vi "ExtraDownsample_4channel.vi"(6 "reset":bool, 7 "Set downsample":bool, 8 "valid in":bool, 9 "Downsample":fxp<+,8,8>, 10 "CIC Gain":fxp<+/-,32,1>=0.00390625 format="%#_32g", 11 "Data in":fxp<+/-,16,14>[](array[numeric])=[0.0, 0.0, 0.0, 0.0, 0.0, 0.0, 0.0, 0.0]) -> (0 "valid out":bool, 3 "Data out":fxp<+/-,16,14>[](array[numeric]))   [LabVIEW 2013]
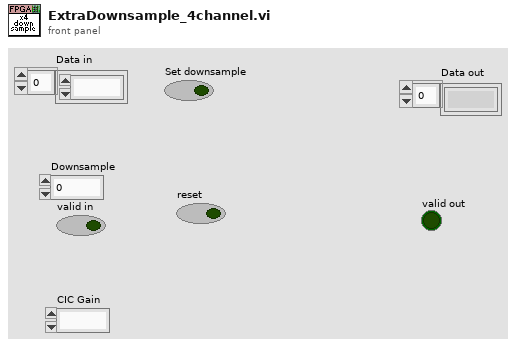
[diagram p1: front panel]
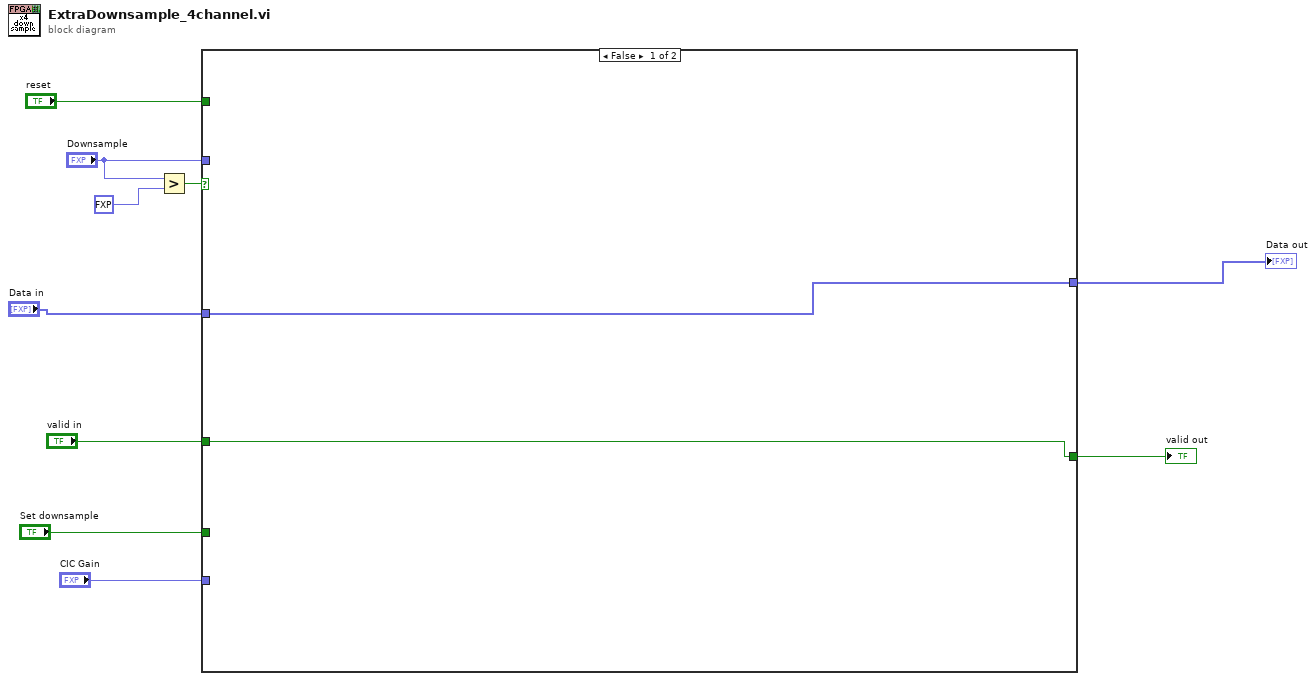
[diagram p0: block diagram]
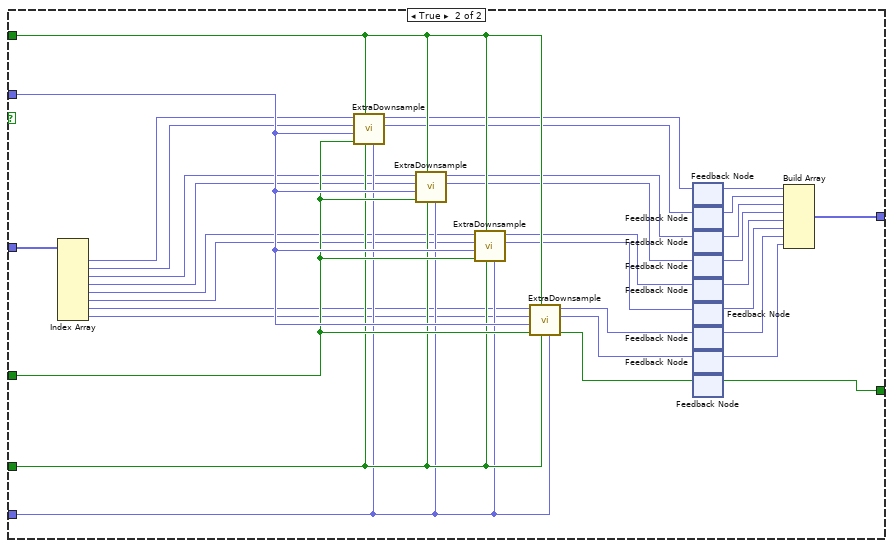
[diagram p2: hidden frame]
diagram:
  n1 = Greater?(x="Downsample", y=fxp<+,8,8> 1.0) -> (0:w2:bool)
  n2 = case shown="False" w2 {
    tunnel: "Data in" -> [w11 w45]
    tunnel: "Downsample" -> [_ w44]
    tunnel: "valid in" -> [w12 w43]
    tunnel: "reset" -> [_ w42]
    tunnel: "Set downsample" -> [_ w41]
    tunnel: "CIC Gain" -> [_ w40]
    tunnel: [w12 w30] -> w3
    tunnel: [w11 w13] -> w1
    frame False {
    }
    frame True {
      n3 = Index Array(array=w45) -> (element #1=w29:fxp<+/-,16,14>, element #2=w28:fxp<+/-,16,14>, element #3=w27:fxp<+/-,16,14>, element #4=w26:fxp<+/-,16,14>, element #5=w25:fxp<+/-,16,14>, element #6=w24:fxp<+/-,16,14>, element #7=w23:fxp<+/-,16,14>, element #8=w22:fxp<+/-,16,14>)  [unwired: 8 in]
      n4 = call "ExtraDownsample.vi"("CIC Gain"=w40, "Set downsample"=w41, "reset"=w42, "valid in"=w43, "Downsample"=w44, "I in"=w28, "Q in"=w29) -> ("Q out"=w38:fxp<+/-,16,14>, "I out"=w39:fxp<+/-,16,14>)  [unwired: 2 in, 1 out]
      n5 = call "ExtraDownsample.vi"("CIC Gain"=w40, "Set downsample"=w41, "reset"=w42, "valid in"=w43, "Downsample"=w44, "I in"=w26, "Q in"=w27) -> ("Q out"=w36:fxp<+/-,16,14>, "I out"=w37:fxp<+/-,16,14>)  [unwired: 2 in, 1 out]
      n6 = call "ExtraDownsample.vi"("CIC Gain"=w40, "Set downsample"=w41, "reset"=w42, "valid in"=w43, "Downsample"=w44, "I in"=w24, "Q in"=w25) -> ("Q out"=w34:fxp<+/-,16,14>, "I out"=w35:fxp<+/-,16,14>)  [unwired: 2 in, 1 out]
      n7 = call "ExtraDownsample.vi"("CIC Gain"=w40, "Set downsample"=w41, "reset"=w42, "valid in"=w43, "Downsample"=w44, "I in"=w22, "Q in"=w23) -> ("valid out"=w31:bool, "Q out"=w32:fxp<+/-,16,14>, "I out"=w33:fxp<+/-,16,14>)  [unwired: 2 in]
      n8 = feedback #1() -> (w21:fxp<+/-,16,14>)  [unwired: 1 in]
      n9 = feedback-in #1(w39) -> ()
      n10 = feedback #2() -> (w20:fxp<+/-,16,14>)  [unwired: 1 in]
      n11 = feedback-in #2(w38) -> ()
      n12 = feedback #3() -> (w19:fxp<+/-,16,14>)  [unwired: 1 in]
      n13 = feedback-in #3(w37) -> ()
      n14 = feedback #4() -> (w18:fxp<+/-,16,14>)  [unwired: 1 in]
      n15 = feedback-in #4(w36) -> ()
      n16 = feedback #5() -> (w17:fxp<+/-,16,14>)  [unwired: 1 in]
      n17 = feedback-in #5(w35) -> ()
      n18 = feedback #6() -> (w16:fxp<+/-,16,14>)  [unwired: 1 in]
      n19 = feedback-in #6(w34) -> ()
      n20 = feedback #7() -> (w15:fxp<+/-,16,14>)  [unwired: 1 in]
      n21 = feedback-in #7(w33) -> ()
      n22 = feedback #8() -> (w14:fxp<+/-,16,14>)  [unwired: 1 in]
      n23 = feedback-in #8(w32) -> ()
      n24 = feedback #9() -> (w30:bool)  [unwired: 1 in]
      n25 = feedback-in #9(w31) -> ()
      n26 = Build Array(w21, w20, w19, w18, w17, w16, w15, w14) -> (w13:fxp<+/-,16,14>[])
    }
  }
  "valid out" <- w3
  "Data out" <- w1
